vi "STM Write Message (Serial).vi"(6 "Options":T1={"Ignore Timeout Error"=TRUE, "timeout ms (1000)"=1000}, 8 "error in (no error)":errorcluster, 9 "Data":string, 10 "Name":string, 11 "Connection Info":T2) -> (0 "error out":errorcluster, 3 "Connection Info Out":T2)   [LabVIEW 2010]
doc: "This VI writes a package of data to a remote computer. It prepends a meta data ID number to each packet. \n\nThe data must be passed in as a String. The calling VI is responsible for flattening the desired data to a string before passing it to this VI. \n\n\nCopyright 2015, 2016, 2017 National Instruments Corporation\n\nLicensed under the Apache License, Version 2.0 (the \"License\"); you may not use this file except in compliance with the License.\n\n You may obtain a copy of the License at\n\n http://www.apache.org/licenses/LICENSE-2.0\n\nUnless required by applicable law or agreed to in writing, software distributed under the License is distributed on an \"AS IS\" BASIS, WITHOUT WARRANTIES OR CONDITIONS OF ANY KIND, either express or implied.\n\nSee the License for the specific language governing permissions and limitations under the License."
uses:
  stm_Serial Connection Info.ctl
  stm_MetaDataElement.ctl
  stm_Serial Write Options.ctl
  NI STM.lvlib
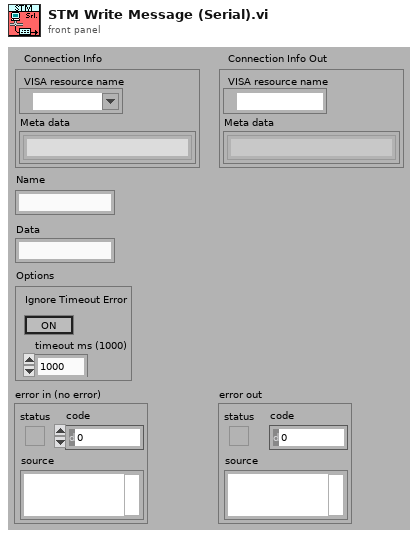
[diagram p1: front panel]
types:
  T1 = typedef "stm_Serial Write Options.ctl" = cluster{"Ignore Timeout Error":bool, "timeout ms (1000)":u32}
  T2 = typedef "stm_Serial Connection Info.ctl" = cluster{"VISA resource name":refnum<visa-resource-name>, "Meta data":T3[]}
  T3 = typedef "stm_MetaDataElement.ctl" = string
  T4 = typedef "NI STM.lvlib/Serial Connection Info.ctl" = cluster{"VISA resource name":refnum<visa-resource-name>, "meta data":T5[]}
  T5 = typedef "NI STM.lvlib/MetaDataElement.ctl" = string
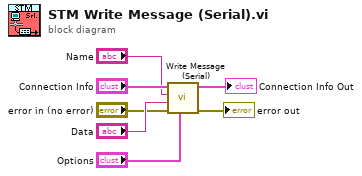
[diagram p0: block diagram]
diagram:
  n1 = call "Write Message (Serial).vi"("options"="Options", "error in"="error in (no error)", "data"="Data", "name"="Name", "connection info in"="Connection Info") -> ("error out"=→"error out":errorcluster, "connection info out"=→"Connection Info Out":T4)  [unwired: 5 in]
